vi "Allvelctrl.vi"(8 "v":dbl=100.0, 10 "dx":dbl=10.0, 15 "dy":dbl) -> (4 "2D Picture":picture, 6 "vq":dbl[](array[numeric]) format="%.2f")   [LabVIEW 2024]
panel:
  out "output cluster":cluster{"L 1":dbl, "L 2":dbl, "q":dbl[]}
  in  "L 2":dbl(slide)=30.0 scale=0.0..200.0
  in  "L 1":dbl(slide)=30.0 scale=0.0..200.0
  in  "bias":dbl
  in  "geometry?":bool=TRUE
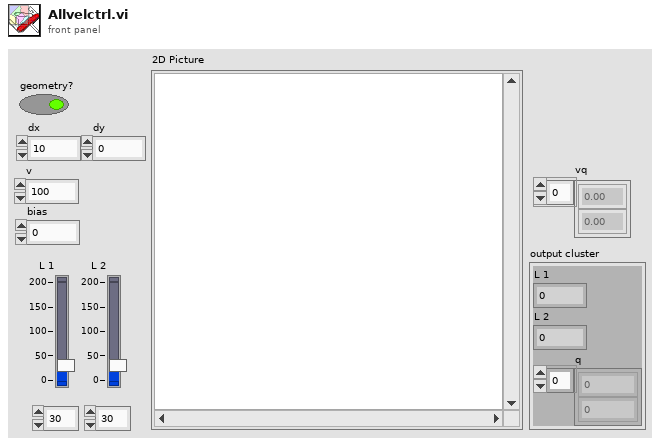
[diagram p1: front panel]
types:
  T1 = cluster{"Width":u16, "Style":enum32{"Solid", "Dash", "Dot", "DashDot", "DashDotDot"}}
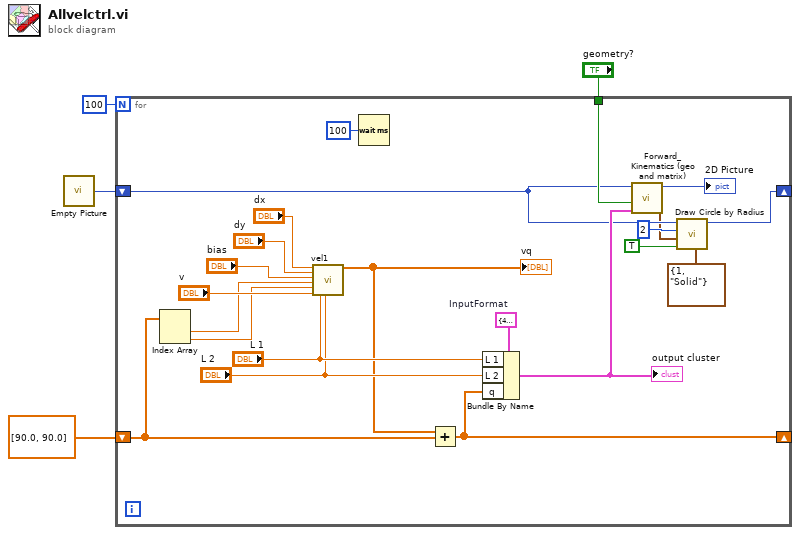
[diagram p0: block diagram]
diagram:
  n1 = call "Empty Picture"() -> ("empty picture"=w1:picture)
  n2 = for {
    N: 100 -> [_]
    tunnel: "geometry?" -> [w19]
    shift-right: [w11] -> _
    shift-left: dbl[] [90.0, 90.0] -> [w14]
    shift-right: [w9] -> _
    shift-left: w1 -> [w7]
    w23 = cluster{"L 1":dbl, "L 2":dbl, "q":dbl[]} {"L 1"=40.0, "L 2"=35.0, "q"=[180.0, 60.0]}  # InputFormat
    n3 = Index Array(array=w14) -> (element #1=w13:dbl, element #2=w12:dbl)  [unwired: 2 in]
    n4 = call "vel1.vi"("dx"="dx", "dy"="dy", "bias"="bias", "Angle1"=w13, "Angle 2"=w12, "v"="v", "L 1"="L 1", "L 2"="L 2") -> ("vq"=w15:dbl[])  [unwired: 10 in, 1 out]
    "vq" <- w15
    n5 = Wait (ms)(milliseconds to wait=u32 100) -> ()  [unwired: 1 out]
    n6 = Add(x=w15, y=w14) -> (x+y=w11:dbl[])
    n7 = Bundle By Name(cluster=w23, "L 1"="L 1", "L 2"="L 2", "q"=w11) -> (w20:cluster{"L 1":dbl, "L 2":dbl, "q":dbl[]})
    "output cluster" <- w20
    n8 = call <userlib>:"Forward_Kinematics (geo and matrix).vi"("geometry"=w20, "geometry?"=w19, "picture in"=w7) -> ("end (2D)"=w6:cluster{"x":dbl, "y":dbl}, "2D Picture"=→"2D Picture":picture)  [unwired: 6 in, 1 out]
    n9 = call <vilib>:"Draw Circle by Radius.vi"("pen"=T1 {"Width"=1, "Style"=enum."Solid"}, "fill?(F)"=TRUE, "pixel center"=w6, "radius"=i16 2, "picture"=w7) -> ("new picture"=w9:picture)  [unwired: 6 in]
  }
